vi "AllFileIO.vi"() -> ()   [LabVIEW 2014]
panel:
  in  "name or relative path":string="FileIO.txt"
  in  "base path":path
  out "text":string
  out "File Name":string
  in  "text to file":string caption="text from file"
  out "Resulting Path":path
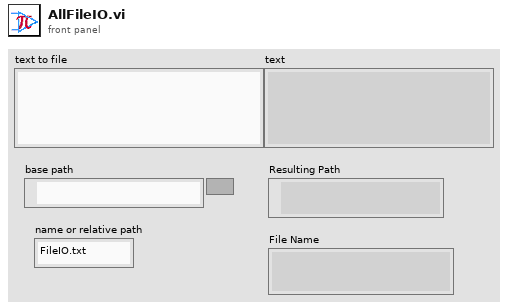
[diagram p1: front panel]
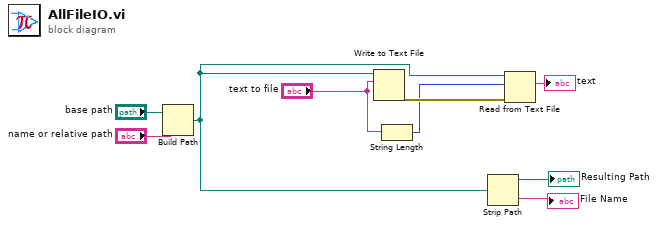
[diagram p0: block diagram]
diagram:
  n1 = Build Path(base path="base path", name or relative path="name or relative path") -> (appended path=w1:path)
  n2 = Write to Text File(file (use dialog)=w1, text="text to file") -> (error out=w5:errorcluster)  [unwired: 2 in, 2 out]
  n3 = String Length(string="text to file") -> (length=w2:i32)
  n4 = Strip Path(path=w1) -> (stripped path=→"Resulting Path":path, name=→"File Name":string)
  n5 = Read from Text File(file (use dialog)=w1, count=w2, error in=w5) -> (text=→"text":string)  [unwired: 1 in, 3 out]
